vi "time2_db.vi"(1 "time stamp":timestamp) -> (0 "date/time string":string)   [LabVIEW 2010]
uses:
  70user.lib/TheSigTab.vi
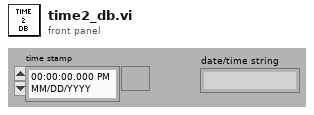
[diagram p1: front panel]
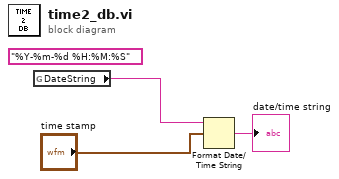
[diagram p0: block diagram]
diagram:
  (unwired) "%Y-%m-%d %H:%M:%S" ("time format string (%c)")
  n1 = global read "TheSigTab.vi" "DateString"() -> (w1:string)
  n2 = Format Date/Time String(time format string (%c)=w1, seconds (now)="time stamp") -> (date/time string=→"date/time string":string)  [unwired: 1 in]
